vi "BBoxLite.vi"() -> ()   [LabVIEW 2022 SP3]
uses:
  D:/tmytek/Source/bbox-api/example/BBoxLite Series/LabVIEW/BBoxAPI.dll
  BBoxAPI.dll
  Kernel32.dll
panel:
  out "Exists Table Filenames":string[](array[string])
  out "Get Current Working Directory":path
  in  "Set Current Working Directory":path
  out "readChannelSwitchValues":i32[][](array[numeric])
  out "setAllChannelGain":i32
  in  "Board_Ch4":dbl
  in  "Board_Ch3":dbl
  in  "Board_Ch2":dbl
  in  "Board_Ch1":dbl
  out "Target AAKit Name":string
  in  "Target AAKit Index":i32 min=1 max=2 step=1
  out "getAAKitList":string[](array[string])
  out "RX Board1 elementDR":dbl
  out "TX Board1 elementDR":dbl
  out "TX Minimum Gain":dbl
  out "TX Maxmum Gain":dbl
  in  "Target Freq Index":i32 min=1 max=2 step=1
  out "setBeamAngle":i32(ring)=13 items=["OK"=0, "WARNING"=1, "ERROR"=2, "NO_RESPONSE"=3, "ERROR_GET_SN"=10, "ERROR_DEV_TYPE"=11, "ERROR_INIT_OBJECT"=12, "ERROR_DEV_NOT_INIT"=13, "ERROR_METHOD_NOT_FOUND"=14, "ERROR_REFLECTION"=15, "ERROR_POWER"=16, "ERROR_NETWORK_NOT_INIT"=20, "ERROR_NETWORK_INIT"=21, "ERROR_NETWORK_CONNECT_TIMEOUT"=22, "ERROR_DISCONNECT"=23, "ERROR_SOCKET"=24, "ERROR_SEND_CMD"=25, "ERROR_RESP_CMD"=26, "ERROR_DEV_COUNT_ZERO"=30, "ERROR_CMD"=40, "ERROR_CMD_INIT"=41, "ERROR_BF_AAKIT"=100, "ERROR_BF_NO_AAKIT"=101, "ERROR_BF_CALI_PATH"=102, "ERROR_BF_BEAMXY"=103, "ERROR_BF_GEN"=104, "ERROR_BF_TRMODE"=105, "STATUS_BF_LOAD_CALI_INCOMPLTE"=106, "ERROR_BF_LOAD_CALI_PARSE_FAILED"=107, "ERROR_FREQ_EQUATION"=250, "ERROR_PLO_CRC"=251, "WARNING_HARMONIC"=252, "ERROR_HARMONIC_BLOCK"=253]
  in  "Phi":i32 min=-45 max=45 step=1
  out "switchChannelPower":string
  in  "Power\nOn = 0\nOff = 1":i32
  out "selectAAKit":i32(ring)=13 items=["OK"=0, "WARNING"=1, "ERROR"=2, "NO_RESPONSE"=3, "ERROR_GET_SN"=10, "ERROR_DEV_TYPE"=11, "ERROR_INIT_OBJECT"=12, "ERROR_DEV_NOT_INIT"=13, "ERROR_METHOD_NOT_FOUND"=14, "ERROR_REFLECTION"=15, "ERROR_POWER"=16, "ERROR_NETWORK_NOT_INIT"=20, "ERROR_NETWORK_INIT"=21, "ERROR_NETWORK_CONNECT_TIMEOUT"=22, "ERROR_DISCONNECT"=23, "ERROR_SOCKET"=24, "ERROR_SEND_CMD"=25, "ERROR_RESP_CMD"=26, "ERROR_DEV_COUNT_ZERO"=30, "ERROR_CMD"=40, "ERROR_CMD_INIT"=41, "ERROR_BF_AAKIT"=100, "ERROR_BF_NO_AAKIT"=101, "ERROR_BF_CALI_PATH"=102, "ERROR_BF_BEAMXY"=103, "ERROR_BF_GEN"=104, "ERROR_BF_TRMODE"=105, "STATUS_BF_LOAD_CALI_INCOMPLTE"=106, "ERROR_BF_LOAD_CALI_PARSE_FAILED"=107, "ERROR_FREQ_EQUATION"=250, "ERROR_PLO_CRC"=251, "WARNING_HARMONIC"=252, "ERROR_HARMONIC_BLOCK"=253]
  out "readBeamPhaseValues":i32[][](array[numeric])
  out "readBeamGainValues":dbl[][](array[numeric])
  in  "Theta":i32=15 min=-45 max=45 step=1
  in  "Beam Gain":dbl step=0.5
  out "setChannelGainPhase":string
  in  "Phase":i32 min=0 max=355 step=5
  in  "Gain":dbl step=0.5
  in  "Channel":i32=1 min=1 max=4
  in  "TxRxMode\nTX = 1\nRx = 2":i32=1 min=1 max=2 step=1
  out "RX Maxmum Gain":dbl
  out "RX Minimum Gain":dbl
  out "getTxRxMode":i32
  out "SwitchTxRxMode":i32(ring) items=["OK"=0, "WARNING"=1, "ERROR"=2, "NO_RESPONSE"=3, "ERROR_GET_SN"=10, "ERROR_DEV_TYPE"=11, "ERROR_INIT_OBJECT"=12, "ERROR_DEV_NOT_INIT"=13, "ERROR_METHOD_NOT_FOUND"=14, "ERROR_REFLECTION"=15, "ERROR_POWER"=16, "ERROR_NETWORK_NOT_INIT"=20, "ERROR_NETWORK_INIT"=21, "ERROR_NETWORK_CONNECT_TIMEOUT"=22, "ERROR_DISCONNECT"=23, "ERROR_SOCKET"=24, "ERROR_SEND_CMD"=25, "ERROR_RESP_CMD"=26, "ERROR_DEV_COUNT_ZERO"=30, "ERROR_CMD"=40, "ERROR_CMD_INIT"=41, "ERROR_BF_AAKIT"=100, "ERROR_BF_NO_AAKIT"=101, "ERROR_BF_CALI_PATH"=102, "ERROR_BF_BEAMXY"=103, "ERROR_BF_GEN"=104, "ERROR_BF_TRMODE"=105, "STATUS_BF_LOAD_CALI_INCOMPLTE"=106, "ERROR_BF_LOAD_CALI_PARSE_FAILED"=107, "ERROR_FREQ_EQUATION"=250, "ERROR_PLO_CRC"=251, "WARNING_HARMONIC"=252, "ERROR_HARMONIC_BLOCK"=253]
  out "setOperatingFreq":i32(ring)=13 items=["OK"=0, "WARNING"=1, "ERROR"=2, "NO_RESPONSE"=3, "ERROR_GET_SN"=10, "ERROR_DEV_TYPE"=11, "ERROR_INIT_OBJECT"=12, "ERROR_DEV_NOT_INIT"=13, "ERROR_METHOD_NOT_FOUND"=14, "ERROR_REFLECTION"=15, "ERROR_POWER"=16, "ERROR_NETWORK_NOT_INIT"=20, "ERROR_NETWORK_INIT"=21, "ERROR_NETWORK_CONNECT_TIMEOUT"=22, "ERROR_DISCONNECT"=23, "ERROR_SOCKET"=24, "ERROR_SEND_CMD"=25, "ERROR_RESP_CMD"=26, "ERROR_DEV_COUNT_ZERO"=30, "ERROR_CMD"=40, "ERROR_CMD_INIT"=41, "ERROR_BF_AAKIT"=100, "ERROR_BF_NO_AAKIT"=101, "ERROR_BF_CALI_PATH"=102, "ERROR_BF_BEAMXY"=103, "ERROR_BF_GEN"=104, "ERROR_BF_TRMODE"=105, "STATUS_BF_LOAD_CALI_INCOMPLTE"=106, "ERROR_BF_LOAD_CALI_PARSE_FAILED"=107, "ERROR_FREQ_EQUATION"=250, "ERROR_PLO_CRC"=251, "WARNING_HARMONIC"=252, "ERROR_HARMONIC_BLOCK"=253]
  out "getFrequencyList":string[](array[string])
  out "Init":i32(ring)=13 items=["OK"=0, "WARNING"=1, "ERROR"=2, "NO_RESPONSE"=3, "ERROR_GET_SN"=10, "ERROR_DEV_TYPE"=11, "ERROR_INIT_OBJECT"=12, "ERROR_DEV_NOT_INIT"=13, "ERROR_METHOD_NOT_FOUND"=14, "ERROR_REFLECTION"=15, "ERROR_POWER"=16, "ERROR_NETWORK_NOT_INIT"=20, "ERROR_NETWORK_INIT"=21, "ERROR_NETWORK_CONNECT_TIMEOUT"=22, "ERROR_DISCONNECT"=23, "ERROR_SOCKET"=24, "ERROR_SEND_CMD"=25, "ERROR_RESP_CMD"=26, "ERROR_DEV_COUNT_ZERO"=30, "ERROR_CMD"=40, "ERROR_CMD_INIT"=41, "ERROR_BF_AAKIT"=100, "ERROR_BF_NO_AAKIT"=101, "ERROR_BF_CALI_PATH"=102, "ERROR_BF_BEAMXY"=103, "ERROR_BF_GEN"=104, "ERROR_BF_TRMODE"=105, "STATUS_BF_LOAD_CALI_INCOMPLTE"=106, "ERROR_BF_LOAD_CALI_PARSE_FAILED"=107, "ERROR_FREQ_EQUATION"=250, "ERROR_PLO_CRC"=251, "WARNING_HARMONIC"=252, "ERROR_HARMONIC_BLOCK"=253]
  out "SN":string
  out "ScanningDevice":string[](array[string])
  # "Notice:\n\nThe Set / Get Current Working Diectory Path must be \nthe sample code directory path\n\nbbox-api\\example\\BBoxLite Series\\LabVIEW\\\n\nand must exist\n\nbbox-api\\example\\BBoxLite Series\\LabVIEW\\BBoxAPI.dll\n\nbbox-api\\example\\BBoxLite Series\\LabVIEW\\files\\\n\nbbox-api\\example\\BBoxLite Series\\LabVIEW\\logs\\\n\n---\n\n1. setChannelGainPhase(int board, int ch, double db, int deg,string sn)\n \n  The formula of channel number(1 ~ 4) :\n\n---\n\n2. setAllChannelGain(int board, double ch1_db,double ch2_db,double ch3_db, double ch4_db, string sn)\n\n  The channel gain settings on the same board should not exceed the board elementDR. \n\n   (1) Example\n           - TX DR = (-5.5 db to 10.5 db) \n           - TX elementDR =   4.5 db\n\n            - Valid Settings :\n               ch1_db = 10.5 db\n               ch2_db = 6 db\n               ch3_db = 10 db\n               ch4_db = 8 db  \n\n\n            - Invalid Settings (ch1_db and ch2_db exceed 4.5 db):\n               ch1_db = 10.5 db\n               ch2_db = 5.5 db\n               ch3_db = 10 db\n               ch4_db = 8 db  \n\n---\n\n3. Channel order on GUI  in labview and TMXLab Kits s different.\n\n\n(1) TMXLAB Kits GUI Channel Order\n\nCh04  Ch03  Ch02  Ch01\n\n\n\n(2) Labview GUI Channel Order\n\nCh01  Ch02  Ch03  Ch04"
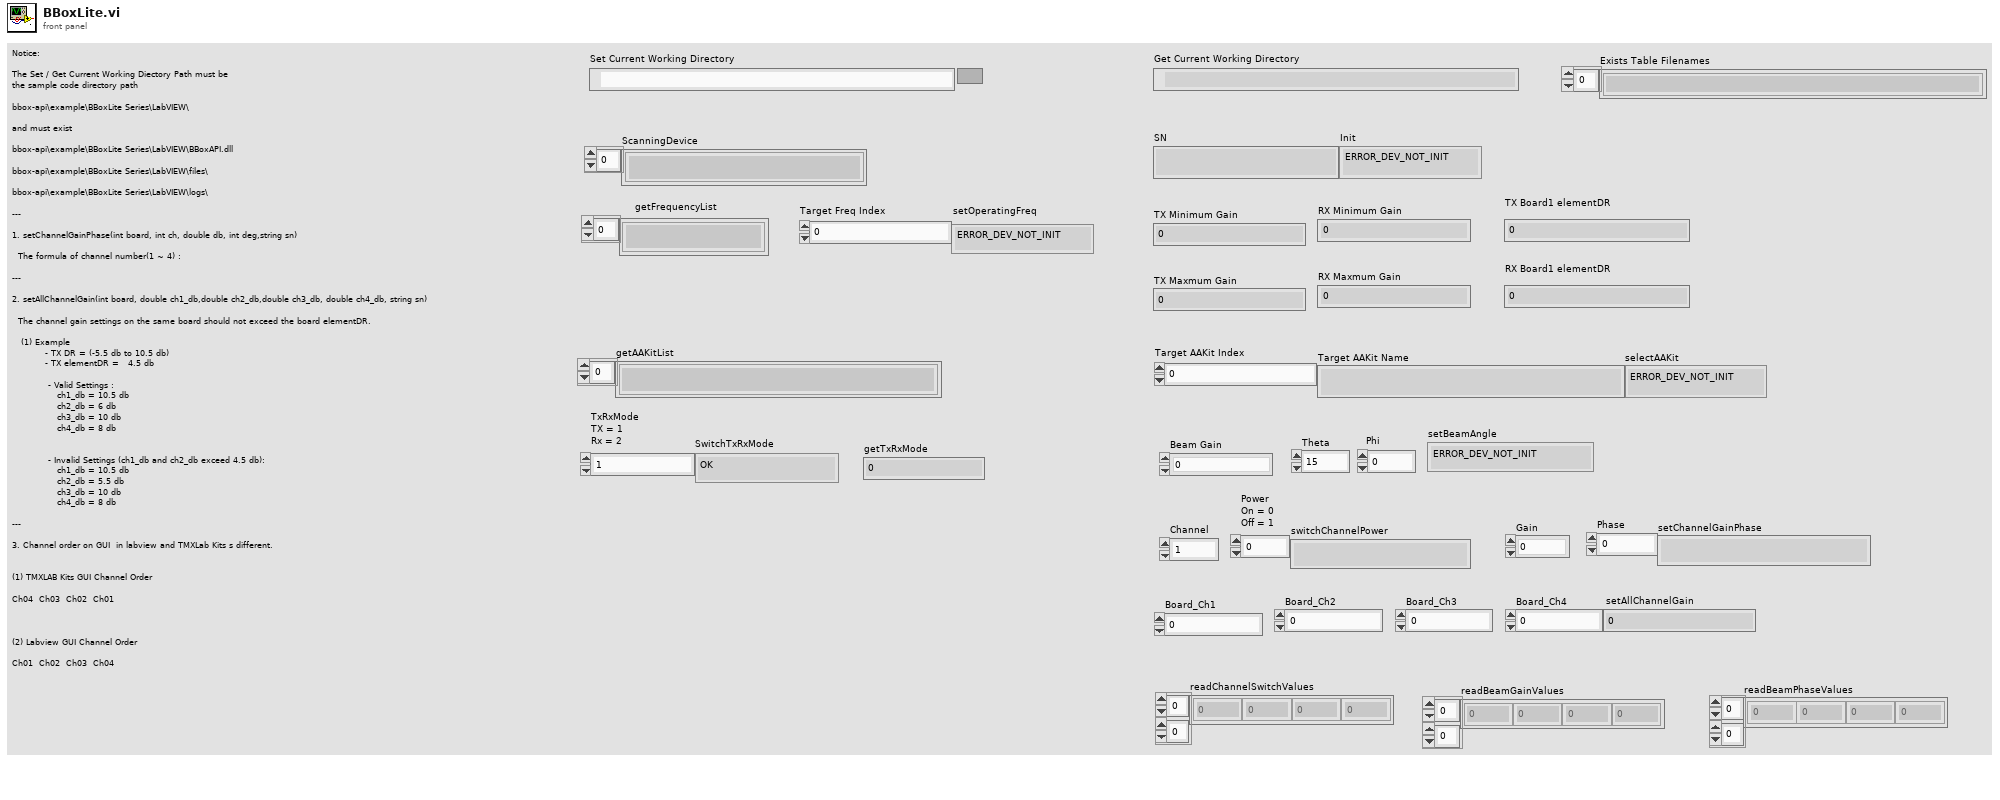
[diagram p1: front panel]
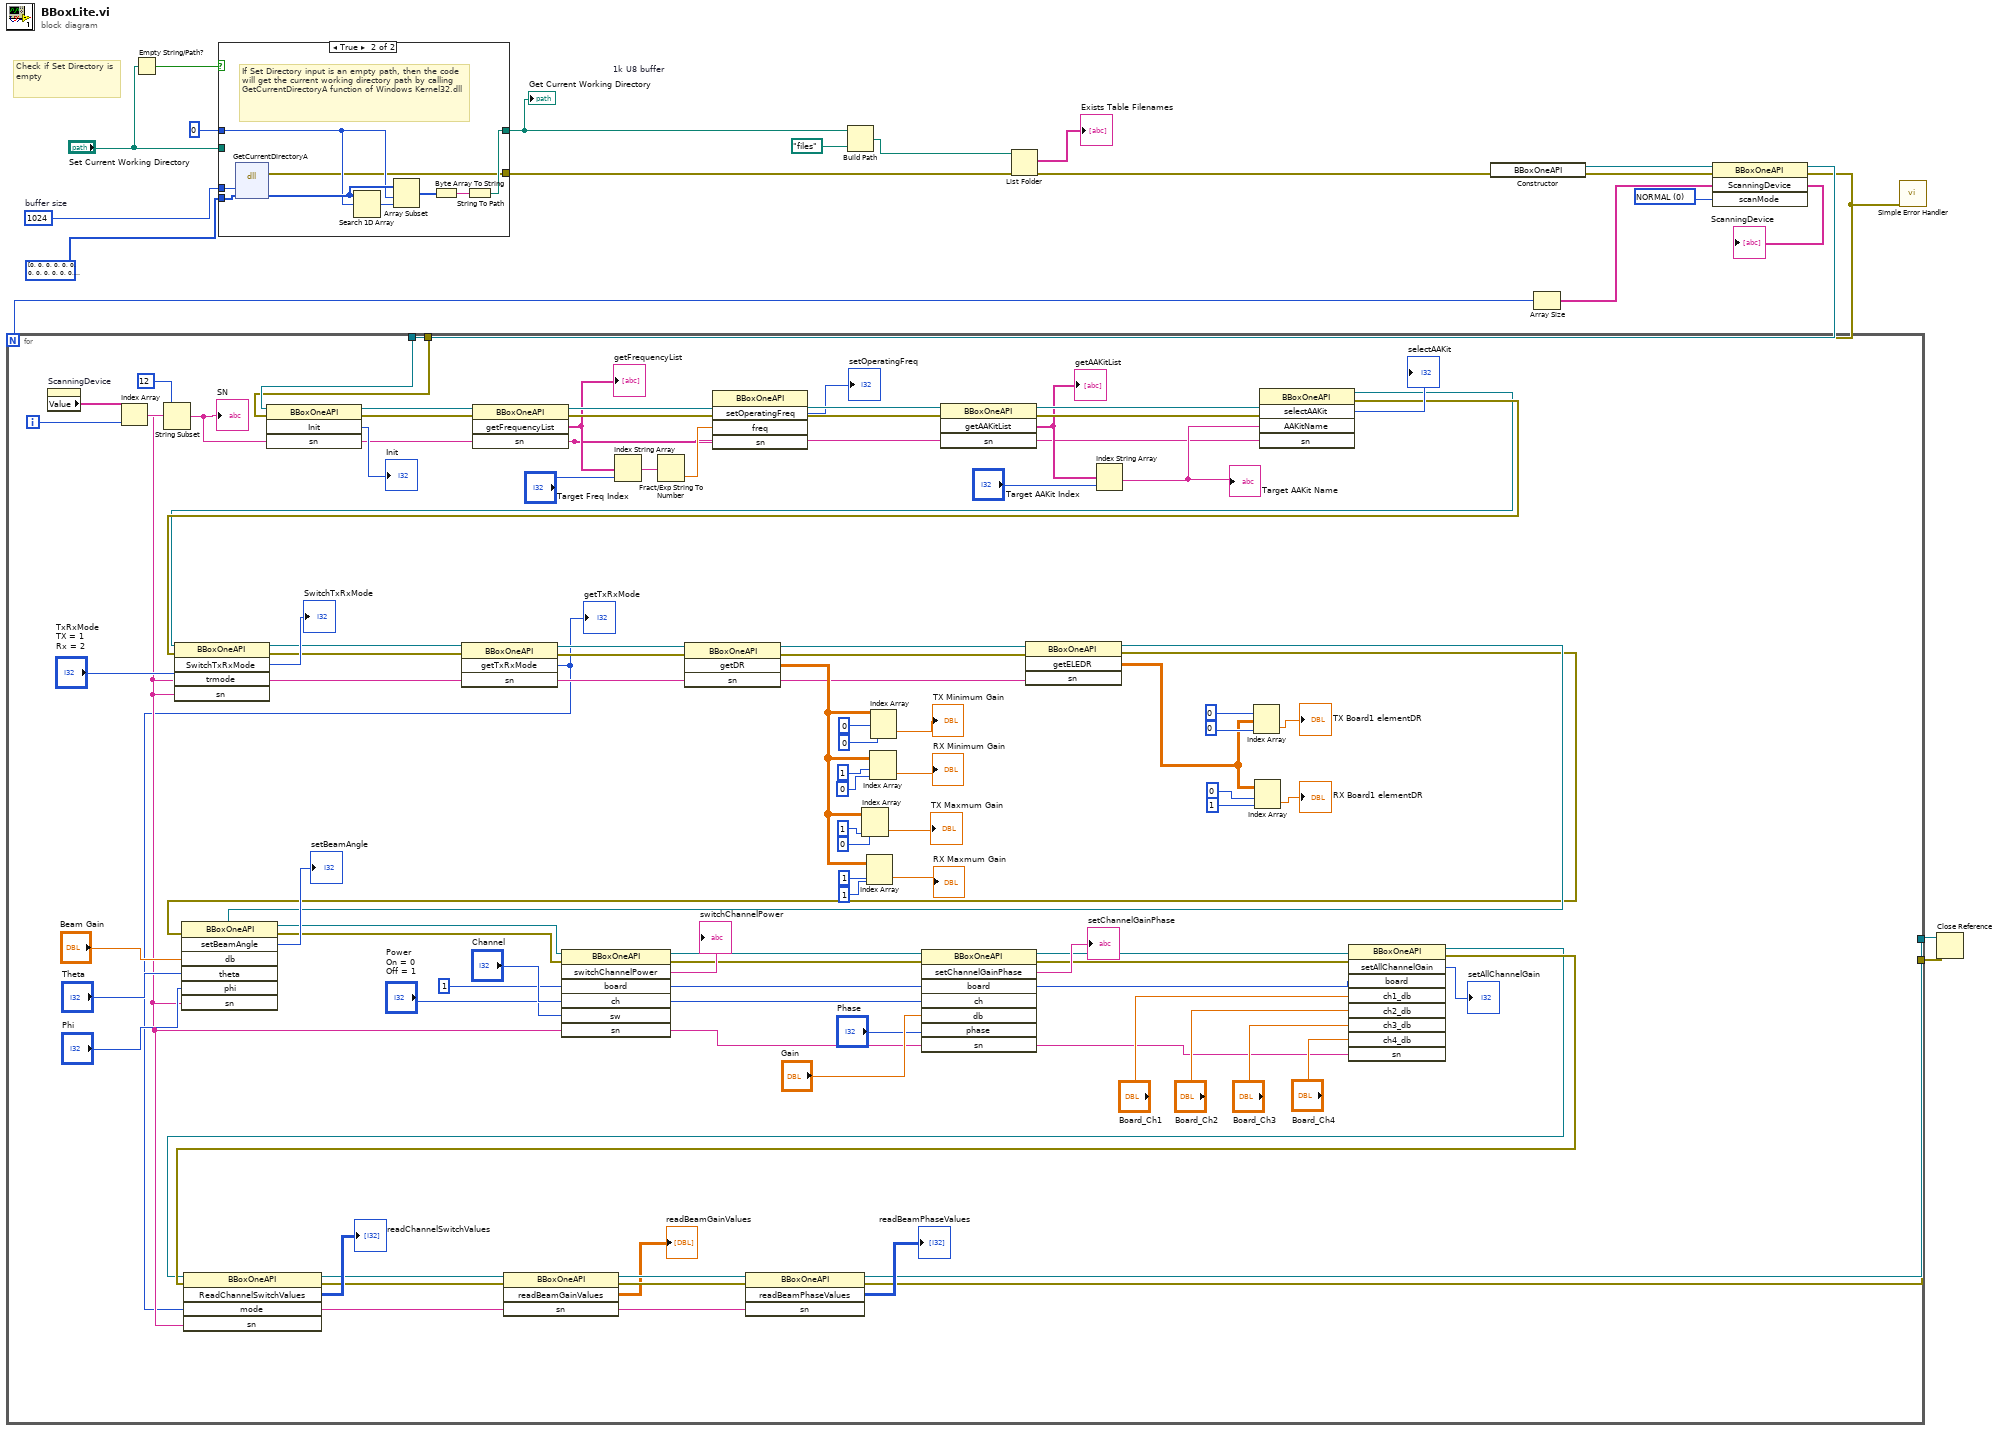
[diagram p0: block diagram]
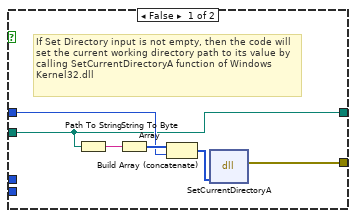
[diagram p2: hidden frame]
diagram:
  w9 = 1024  # buffer size
  w8 = u8[] [0, 0, 0, 0, 0, 0, 0, 0, 0, 0, 0, 0, 0, 0, 0, 0, 0, 0, 0, 0, 0, 0, 0, 0, 0, 0, 0, 0, 0, 0, 0, 0, 0, 0, 0, 0, 0, 0, 0, 0, 0, 0, 0, 0, 0, 0, 0, 0, 0, 0, 0, 0, 0, 0, 0, 0, 0, 0, 0, 0, 0, 0, 0, 0, 0, 0, 0, 0, 0, 0, 0, 0, 0, 0, 0, 0, 0, 0, 0, 0, 0, 0, 0, 0, 0, 0, 0, 0, 0, 0, 0, 0, 0, 0, 0, 0, 0, 0, 0, 0, 0, 0, 0, 0, 0, 0, 0, 0, 0, 0, 0, 0, 0, 0, 0, 0, 0, 0, 0, 0, 0, 0, 0, 0, 0, 0, 0, 0, 0, 0, 0, 0, 0, 0, 0, 0, 0, 0, 0, 0, 0, 0, 0, 0, 0, 0, 0, 0, 0, 0, 0, 0, 0, 0, 0, 0, 0, 0, 0, 0, 0, 0, 0, 0, 0, 0, 0, 0, 0, 0, 0, 0, 0, 0, 0, 0, 0, 0, 0, 0, 0, 0, 0, 0, 0, 0, 0, 0, 0, 0, 0, 0, 0, 0, 0, 0, 0, 0, 0, 0, 0, 0, 0, 0, 0, 0, 0, 0, 0, 0, 0, 0, 0, 0, 0, 0, 0, 0, 0, 0, 0, 0, 0, 0, 0, 0, 0, 0, 0, 0, 0, 0, 0, 0, 0, 0, 0, 0, 0, 0, 0, 0, 0, 0, 0, 0, 0, 0, 0, 0, 0, 0, 0, 0, 0, 0, 0, 0, 0, 0, 0, 0, 0, 0, 0, 0, 0, 0, 0, 0, 0, 0, 0, 0, 0, 0, 0, 0, 0, 0, 0, 0, 0, 0, 0, 0, 0, 0, 0, 0, 0, 0, 0, 0, 0, 0, 0, 0, 0, 0, 0, 0, 0, 0, 0, 0, 0, 0, 0, 0, 0, 0, 0, 0, 0, 0, 0, 0, 0, 0, 0, 0, 0, 0, 0, 0, 0, 0, 0, 0, 0, 0, 0, 0, 0, 0, 0, 0, 0, 0, 0, 0, 0, 0, 0, 0, 0, 0, 0, 0, 0, 0, 0, 0, 0, 0, 0, 0, 0, 0, 0, 0, 0, 0, 0, 0, 0, 0, 0, 0, 0, 0, 0, 0, 0, 0, 0, 0, 0, 0, 0, 0, 0, 0, 0, 0, 0, 0, 0, 0, 0, 0, 0, 0, 0, 0, 0, 0, 0, 0, 0, 0, 0, 0, 0, 0, 0, 0, 0, 0, 0, 0, 0, 0, 0, 0, 0, 0, 0, 0, 0, 0, 0, 0, 0, 0, 0, 0, 0, 0, 0, 0, 0, 0, 0, 0, 0, 0, 0, 0, 0, 0, 0, 0, 0, 0, 0, 0, 0, 0, 0, 0, 0, 0, 0, 0, 0, 0, 0, 0, 0, 0, 0, 0, 0, 0, 0, 0, 0, 0, 0, 0, 0, 0, 0, 0, 0, 0, 0, 0, 0, 0, 0, 0, 0, 0, 0, 0, 0, 0, 0, 0, 0, 0, 0, 0, 0, 0, 0, 0, 0, 0, 0, 0, 0, 0, 0, 0, 0, 0, 0, 0, 0, 0, 0, 0, 0, 0, 0, 0, 0, 0, 0, 0, 0, 0, 0, 0, 0, 0, 0, 0, 0, 0, 0, 0, 0, 0, 0, 0, 0, 0, 0, 0, 0, 0, 0, 0, 0, 0, 0, 0, 0, 0, 0, 0, 0, 0, 0, 0, 0, 0, 0, 0, 0, 0, 0, 0, 0, 0, 0, 0, 0, 0, 0, 0, 0, 0, 0, 0, 0, 0, 0, 0, 0, 0, 0, 0, 0, 0, 0, 0, 0, 0, 0, 0, 0, 0, 0, 0, 0, 0, 0, 0, 0, 0, 0, 0, 0, 0, 0, 0, 0, 0, 0, 0, 0, 0, 0, 0, 0, 0, 0, 0, 0, 0, 0, 0, 0, 0, 0, 0, 0, 0, 0, 0, 0, 0, 0, 0, 0, 0, 0, 0, 0, 0, 0, 0, 0, 0, 0, 0, 0, 0, 0, 0, 0, 0, 0, 0, 0, 0, 0, 0, 0, 0, 0, 0, 0, 0, 0, 0, 0, 0, 0, 0, 0, 0, 0, 0, 0, 0, 0, 0, 0, 0, 0, 0, 0, 0, 0, 0, 0, 0, 0, 0, 0, 0, 0, 0, 0, 0, 0, 0, 0, 0, 0, 0, 0, 0, 0, 0, 0, 0, 0, 0, 0, 0, 0, 0, 0, 0, 0, 0, 0, 0, 0, 0, 0, 0, 0, 0, 0, 0, 0, 0, 0, 0, 0, 0, 0, 0, 0, 0, 0, 0, 0, 0, 0, 0, 0, 0, 0, 0, 0, 0, 0, 0, 0, 0, 0, 0, 0, 0, 0, 0, 0, 0, 0, 0, 0, 0, 0, 0, 0, 0, 0, 0, 0, 0, 0, 0, 0, 0, 0, 0, 0, 0, 0, 0, 0, 0, 0, 0, 0, 0, 0, 0, 0, 0, 0, 0, 0, 0, 0, 0, 0, 0, 0, 0, 0, 0, 0, 0, 0, 0, 0, 0, 0, 0, 0, 0, 0, 0, 0, 0, 0, 0, 0, 0, 0, 0, 0, 0, 0, 0, 0, 0, 0, 0, 0, 0, 0, 0, 0, 0, 0, 0, 0, 0, 0, 0, 0, 0, 0, 0, 0, 0, 0, 0, 0, 0, 0, 0, 0, 0, 0, 0, 0, 0, 0, 0, 0, 0, 0, 0, 0, 0, 0, 0, 0, 0, 0, 0, 0, 0, 0, 0, 0, 0, 0, 0, 0, 0, 0, 0, 0, 0, 0, 0, 0, 0, 0, 0, 0, 0, 0, 0, 0, 0, 0, 0, 0, 0, 0, 0, 0, 0, 0, 0, 0, 0, 0, 0, 0, 0, 0, 0, 0, 0, 0, 0, 0, 0, 0, 0, 0, 0, 0, 0, 0, 0, 0, 0, 0, 0, 0, 0, 0, 0, 0, 0, 0, 0, 0, 0, 0, 0, 0, 0, 0, 0, 0, 0, 0, 0, 0, 0, 0, 0, 0, 0, 0, 0, 0, 0, 0, 0, 0, 0, 0, 0, 0, 0, 0, 0, 0, 0, 0, 0, 0, 0, 0, 0, 0, 0, 0, 0, 0, 0, 0, 0, 0, 0, 0, 0, 0, 0, 0, 0, 0, 0, 0, 0, 0, 0, 0, 0, 0, 0, 0, 0, 0, 0]  # 1k U8 buffer
  w20 = 0 items=["NORMAL", "FAST"] ("scanMode")
  # "Check if Set Directory is empty"
  n1 = Empty String/Path?(string/path="Set Current Working Directory") -> (empty?=w10:bool)
  n2 = case shown="True" w10 {
    tunnel: "Set Current Working Directory" -> [w22 _]
    tunnel: u8 0 -> [w24 w31]
    tunnel: w9 -> [_ w30]
    tunnel: w8 -> [_ w29]
    tunnel: [w22 w28] -> w3
    tunnel: [w21 w27] -> w2
    frame False {
      # "If Set Directory input is not empty, then the code will set the current working directory path to its value by calling SetCurrentDirectoryA function of Windows Kernel32.dll"
      n3 = Path To String(path=w22) -> (string=w23:string)
      n4 = String To Byte Array(string=w23) -> (unsigned byte array=w26:u8[])
      n5 = Build Array (concatenate)(w26, w24) -> (w25:u8[])
      n6 = dll-call lib="Kernel32.dll" fn="SetCurrentDirectoryA" label="Kernel32.dll - \nSetCurrentDirectoryA"("lpPathName"=w25) -> (error out=w21:errorcluster)  [unwired: 4 in, 2 out]
    }
    frame True {
      # "If Set Directory input is an empty path, then the code will get the current working directory path by calling GetCurrentDirectoryA function of Windows Kernel32.dll"
      n7 = dll-call lib="kernel32.dll" fn="GetCurrentDirectoryA" label="Kernel32.dll - \nGetCurrentDirectoryA"("nBufferLength"=w30, "lpBuffer"=w29) -> (error out=w27:errorcluster, "lpBuffer"=w34:u8[])  [unwired: 4 in, 2 out]
      n8 = Search 1D Array(1D array=w34, element=w31) -> (index of element=w35:i32)  [unwired: 1 out]
      n9 = Array Subset(array=w34, index=w31, length=w35) -> (w32:u8[])
      n10 = Byte Array To String(unsigned byte array=w32) -> (string=w33:string)
      n11 = String To Path(string=w33) -> (path=w28:path)
    }
  }
  "Get Current Working Directory" <- w3
  n12 = Build Path(base path=w3, name or relative path=path "files") -> (appended path=w4:path)
  n13 = List Folder(path=w4, error in=w2) -> (filenames=→"Exists Table Filenames":string[], error out=w1:errorcluster)  [unwired: 2 in, 2 out]
  n14 = constructor class="BBoxOneAPI"(error in=w1) -> (reference out=w19:refnum<k24>, error out=w18:errorcluster)  [unwired: 2 in, 1 out]
  n15 = invoke class="BBoxOneAPI" method="ScanningDevice"(reference=w19, error in=w18, "scanMode"=w20) -> (reference out=w15:refnum<k24>, error out=w14:errorcluster, "ScanningDevice"=w16:string[])  [unwired: 1 in, 1 out]
  "ScanningDevice" <- w16
  n16 = Array Size(array=w16) -> (size(s)=w17:i32)
  n17 = for {
    N: w17 -> [_]
    tunnel: w15 -> [w124]
    tunnel: w14 -> [w123]
    tunnel: [w37] -> w13
    tunnel: [w38] -> w12
    i -> [w83]
    w52 = 1
    n18 = property on="ScanningDevice" class="Arr (strict)"() -> ("Value"=w89:string[])  [unwired: 2 in, 2 out]
    n19 = Index Array(array=w89, index=w83) -> (element=w126:string)
    n20 = String Subset(string=w126, length (rest)=12) -> (substring=w41:string)  [unwired: 1 in]
    "SN" <- w41
    n21 = invoke class="BBoxOneAPI" method="Init"(reference=w124, error in=w123, "sn"=w41) -> (reference out=w88:refnum<k24>, error out=w87:errorcluster, "Init"=→"Init":i32)  [unwired: 1 in, 1 out]
    n22 = invoke class="BBoxOneAPI" method="getFrequencyList"(reference=w88, error in=w87, "sn"=w41) -> (reference out=w86:refnum<k24>, error out=w85:errorcluster, "getFrequencyList"=w79:string[])  [unwired: 1 in, 1 out]
    "getFrequencyList" <- w79
    n23 = Index String Array(1:"Target Freq Index", 2:w79) -> (0:w77:string)  [unwired: 1 in]
    n24 = Fract/Exp String To Number(string=w77) -> (number=w76:dbl)  [unwired: 3 in, 1 out]
    n25 = invoke class="BBoxOneAPI" method="setOperatingFreq"(reference=w86, error in=w85, "freq"=w76, "sn"=w41) -> (reference out=w93:refnum<k24>, error out=w92:errorcluster, "setOperatingFreq"=→"setOperatingFreq":i32)  [unwired: 1 in, 2 out]
    n26 = invoke class="BBoxOneAPI" method="getAAKitList"(reference=w93, error in=w92, "sn"=w41) -> (reference out=w91:refnum<k24>, error out=w90:errorcluster, "getAAKitList"=w63:string[])  [unwired: 1 in, 1 out]
    "getAAKitList" <- w63
    n27 = Index String Array(1:"Target AAKit Index", 2:w63) -> (0:w61:string)  [unwired: 1 in]
    "Target AAKit Name" <- w61
    n28 = invoke class="BBoxOneAPI" method="selectAAKit"(reference=w91, error in=w90, "AAKitName"=w61, "sn"=w41) -> (reference out=w81:refnum<k24>, error out=w82:errorcluster, "selectAAKit"=→"selectAAKit":i32)  [unwired: 1 in, 2 out]
    n29 = invoke class="BBoxOneAPI" method="SwitchTxRxMode"(reference=w81, error in=w82, "trmode"="TxRxMode\nTX = 1\nRx = 2", "sn"=w41) -> (reference out=w120:refnum<k24>, error out=w119:errorcluster, "SwitchTxRxMode"=→"SwitchTxRxMode":i32)  [unwired: 1 in, 2 out]
    n30 = invoke class="BBoxOneAPI" method="getTxRxMode"(reference=w120, error in=w119, "sn"=w41) -> (reference out=w118:refnum<k24>, error out=w117:errorcluster, "getTxRxMode"=w36:i32)  [unwired: 1 in, 1 out]
    "getTxRxMode" <- w36
    n31 = invoke class="BBoxOneAPI" method="getDR"(reference=w118, error in=w117, "sn"=w41) -> (reference out=w64:refnum<k24>, error out=w65:errorcluster, "getDR"=w110:dbl[][])  [unwired: 1 in, 1 out]
    n32 = Index Array(array=w110, index (row)=0, index (col)=1) -> (element=→"TX Maxmum Gain":dbl)
    n33 = Index Array(array=w110, index (row)=1, index (col)=1) -> (element=→"RX Maxmum Gain":dbl)
    n34 = Index Array(array=w110, index (row)=1, index (col)=0) -> (element=→"RX Minimum Gain":dbl)
    n35 = Index Array(array=w110, index (row)=0, index (col)=0) -> (element=→"TX Minimum Gain":dbl)
    n36 = invoke class="BBoxOneAPI" method="getELEDR"(reference=w64, error in=w65, "sn"=w41) -> (reference out=w59:refnum<k24>, error out=w58:errorcluster, "getELEDR"=w60:dbl[][])  [unwired: 1 in, 1 out]
    n37 = invoke class="BBoxOneAPI" method="setBeamAngle"(reference=w59, error in=w58, "db"="Beam Gain", "theta"="Theta", "phi"="Phi", "sn"=w41) -> (reference out=w56:refnum<k24>, error out=w55:errorcluster, "setBeamAngle"=→"setBeamAngle":i32)  [unwired: 1 in, 4 out]
    n38 = invoke class="BBoxOneAPI" method="switchChannelPower"(reference=w56, error in=w55, "board"=w52, "ch"="Channel", "sw"="Power\nOn = 0\nOff = 1", "sn"=w41) -> (reference out=w54:refnum<k24>, error out=w53:errorcluster, "switchChannelPower"=→"switchChannelPower":string)  [unwired: 1 in, 4 out]
    n39 = invoke class="BBoxOneAPI" method="setChannelGainPhase"(reference=w54, error in=w53, "board"=w52, "ch"="Channel", "db"="Gain", "phase"="Phase", "sn"=w41) -> (reference out=w46:refnum<k24>, error out=w45:errorcluster, "setChannelGainPhase"=→"setChannelGainPhase":string)  [unwired: 1 in, 5 out]
    n40 = Index Array(array=w60, index (row)=0, index (col)=0) -> (element=→"TX Board1 elementDR":dbl)
    n41 = Index Array(array=w60, index (row)=0, index (col)=1) -> (element=→"RX Board1 elementDR":dbl)
    n42 = invoke class="BBoxOneAPI" method="setAllChannelGain"(reference=w46, error in=w45, "board"=w52, "ch1_db"="Board_Ch1", "ch2_db"="Board_Ch2", "ch3_db"="Board_Ch3", "ch4_db"="Board_Ch4", "sn"=w41) -> (reference out=w39:refnum<k24>, error out=w40:errorcluster, "setAllChannelGain"=→"setAllChannelGain":i32)  [unwired: 1 in, 6 out]
    n43 = invoke class="BBoxOneAPI" method="ReadChannelSwitchValues"(reference=w39, error in=w40, "mode"=w36, "sn"=w41) -> (reference out=w43:refnum<k24>, error out=w42:errorcluster, "ReadChannelSwitchValues"=→"readChannelSwitchValues":i32[][])  [unwired: 1 in, 2 out]
    n44 = invoke class="BBoxOneAPI" method="readBeamGainValues"(reference=w43, error in=w42, "sn"=w41) -> (reference out=w101:refnum<k24>, error out=w100:errorcluster, "readBeamGainValues"=→"readBeamGainValues":dbl[][])  [unwired: 1 in, 1 out]
    n45 = invoke class="BBoxOneAPI" method="readBeamPhaseValues"(reference=w101, error in=w100, "sn"=w41) -> (reference out=w38:refnum<k24>, error out=w37:errorcluster, "readBeamPhaseValues"=→"readBeamPhaseValues":i32[][])  [unwired: 1 in, 1 out]
  }
  n46 = call <vilib>:"Simple Error Handler.vi"("error in (no error)"=w14) -> ()  [unwired: 4 in, 5 out]
  n47 = Close Reference(reference=w12, error in (no error)=w13) -> ()  [unwired: 1 out]
